vi "time loop servo control.vi"() -> ()   [LabVIEW 2022 SP3]
uses:
  <vilib>/Platform/TimedLoop/XDataNode/timing_clust.ctl
  <vilib>/Platform/TimedLoop/XDataNode/nitl_modes.ctl
  <vilib>/Platform/TimedLoop/XDataNode/wakeup.ctl
  <vilib>/DAQmx/write.llb/DAQmx Write (Digital Bool 1Line 1Point).vi
  <vilib>/DAQmx/create/channels.llb/DAQmx Create Channel (DO-Digital Output).vi
  <vilib>/Platform/TimedLoop/TimeConversion.llb/rt-rel-time-to-milliseconds.vi
  <vilib>/DAQmx/miscellaneous.llb/DAQmx Fill In Error Info.vi
  <vilib>/platform/TimedLoop/XDataNode/XDataNode.xnode
  <vilib>/Platform/TimedLoop/XDataNode/XDNodeRunTimeDep.lvlib
panel:
  in  "stop":bool
  in  "lines 2":tag
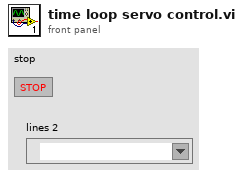
[diagram p1: front panel]
types:
  T1 = typedef "XDNodeRunTimeDep.lvlib/timing_clust.ctl" = cluster{"Expected End [f-1]":u64, "Actual End [f-1]":u64, "Finished Late? [f-1]":bool, "Expected End [i-1]":u64, "Actual End [i-1]":u64, "Finished Late? [i-1]":bool, "Expected Start [i]":u64, "Actual Start [i]":u64, "Expected Start [f]":u64, "Actual Start [f]":u64, "Source Name":string, "Structure Name":string, "Period":i64, "Deadline":i64, "Offset":i64, "Start":i64, "Priority":i32, "Timeout":i32, "Mode":T2, "Wakeup Reason":T3, "Error":errorcluster, "Source Type":string, "Secondary Source Type":string, "Global End Time":u64, "Global Start Time":u64, "Frame Duration":u64, "Iteration Duration":u64, "Assigned CPU":i32, "I/O Scan Engine Mode":u32}
  T2 = typedef "XDNodeRunTimeDep.lvlib/nitl_modes.ctl" = enum32{"No Change", "Process missed periods, maintain original phase", "Discard missed periods, maintain original phase", "Process missed periods, ignore original phase", "Discard missed periods, ignore original phase"}
  T3 = typedef "XDNodeRunTimeDep.lvlib/wakeup.ctl" = enum32{"Normal", "Aborted", "Asynchronous wakeup", "Timing source error", "Timed loop error", "Timeout"}
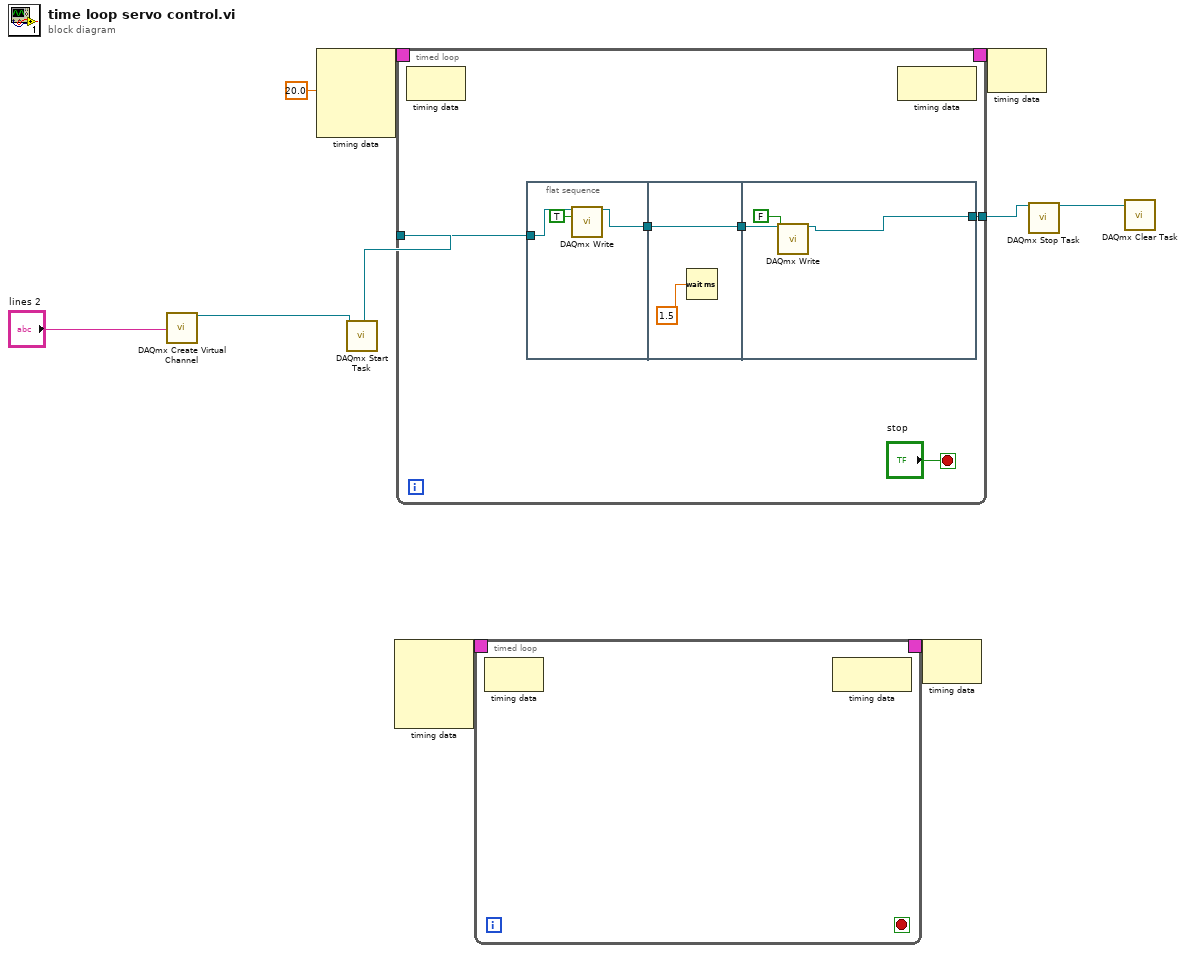
[diagram p0: block diagram]
diagram:
  n1 = call-poly <vilib>:"DAQmx Create Virtual Channel.vi"("lines"="lines 2") -> ("task out"=w9:refnum<k21>)  [unwired: 13 in, 1 out]
  n2 = node-c288(20.0 ("Period")) -> (w5:T1)  [unwired: 3 in]
  n3 = call <vilib>:"DAQmx Start Task.vi"("task/channels in"=w9) -> ("task out"=w8:refnum<k21>)  [unwired: 13 in, 1 out]
  n4 = node-c288() -> (w3:T1)  [unwired: 4 in]
  n5 = timed-loop {
    tunnel: w8 -> [w15]
    tunnel: [w12] -> w6
    timing: w5 -> [_]
    timing-out: [_] -> w4
    stop <- "stop" stop-if-true
    n6 = node-c288() -> ()  [unwired: 1 in, 1 out]
    n7 = flat-sequence {
      tunnel: w15 -> [w20]
      tunnel: [w19] -> w13
      tunnel: [w22] -> w14
      tunnel: w13 -> [w22]
      tunnel: [w25] -> w12
      tunnel: w14 -> [w24]
      frame #0 {
        n8 = call-poly <vilib>:"DAQmx Write.vi"("task/channels in"=w20, "data"=TRUE) -> ("task out"=w19:refnum<k21>)  [unwired: 11 in, 2 out]
      }
      frame #1 {
        n9 = Wait (ms)(milliseconds to wait=1.5) -> ()  [unwired: 1 out]
      }
      frame #2 {
        n10 = call-poly <vilib>:"DAQmx Write.vi"("task/channels in"=w24, "data"=FALSE) -> ("task out"=w25:refnum<k21>)  [unwired: 11 in, 2 out]
      }
    }
    n11 = node-c288() -> ()  [unwired: 1 in, 1 out]
  }
  n12 = timed-loop {
    timing: w3 -> [_]
    timing-out: [_] -> w2
    stop <- _ stop-if-true
    n13 = node-c288() -> ()  [unwired: 1 in, 1 out]
    n14 = node-c288() -> ()  [unwired: 1 in, 1 out]
  }
  n15 = node-c288(w2) -> ()  [unwired: 1 out]
  n16 = node-c288(w4) -> ()  [unwired: 1 out]
  n17 = call <vilib>:"DAQmx Stop Task.vi"("task/channels in"=w6) -> ("task out"=w7:refnum<k21>)  [unwired: 13 in, 1 out]
  n18 = call <vilib>:"DAQmx Clear Task.vi"("task in"=w7) -> ()  [unwired: 14 in, 1 out]
